vi "Find attached USB cameras.vi"() -> ()   [LabVIEW 2025]
uses:
  <vilib>/userDefined/High Color/IMAQdx.ctl
  <vilib>/nisyscfg/nisyscfg.lvlib
  <resource>/objmgr/nicriosae.rc
  <vilib>/vision/driver/NI_Vision_Acquisition_Software.lvlib
  <resource>/objmgr/imaqdx.rc
panel:
  out "map":map{u32, T1}(c390)
  out "Serial Number":u32[](array[numeric])
  out "Product":string[](array[string])
  out "Camera":string[](array[string])
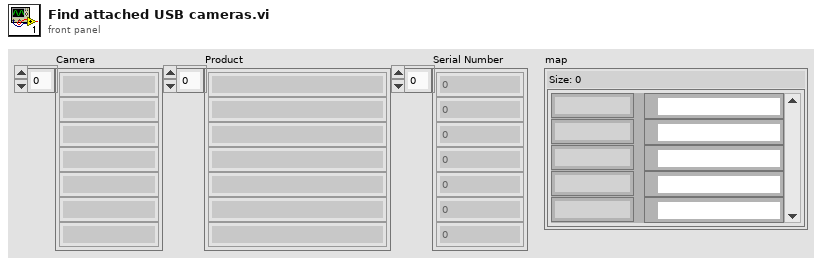
[diagram p1: front panel]
types:
  T1 = typedef "IMAQdx.ctl" = refnum<k21>
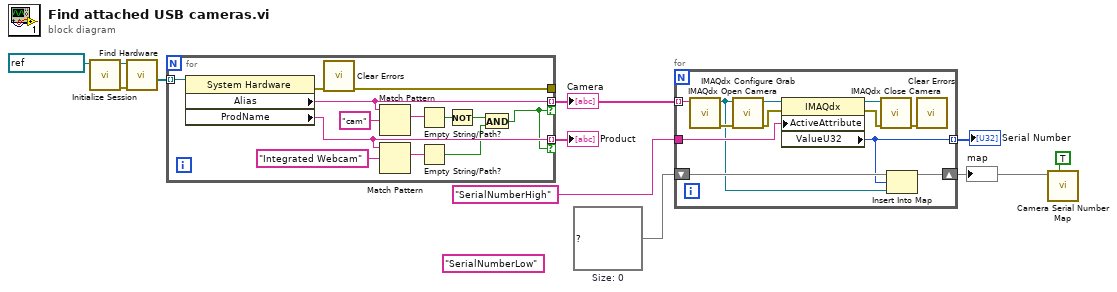
[diagram p0: block diagram]
diagram:
  w4 = map{u32, T1} {}  # Size: 0
  (unwired) "SerialNumberLow"
  n1 = call <vilib>:"Initialize Session.vi"("Target (localhost)"=refnum<k21> "localhost") -> ("error out"=w10:errorcluster, "Session out"=w11:refnum<k21>)  [unwired: 9 in]
  n2 = call <vilib>:"Find Hardware.vi"("error in (no error)"=w10, "Session in"=w11) -> ("Resources out"=w8:refnum<k20>[])  [unwired: 6 in, 3 out]
  n3 = for {
    tunnel: w8 -> [w24] mode=indexing
    tunnel: [w16] -> w7 mode=indexing if=w12
    tunnel: [w22] -> _
    tunnel: [w21] -> w6 mode=indexing if=w12
    n4 = property class="System Hardware"(reference=w24) -> (error out=w23:errorcluster, "Alias"=w21:string, "ProdName"=w16:string)  [unwired: 1 in, 1 out]
    n5 = call <vilib>:"Clear Errors.vi"("error in (no error)"=w23) -> ("error out"=w22:errorcluster)  [unwired: 5 in, 1 out]
    n6 = Match Pattern(string=w21, regular expression="cam") -> (match substring=w19:string)  [unwired: 1 in, 3 out]
    n7 = Match Pattern(string=w16, regular expression="Integrated Webcam") -> (match substring=w15:string)  [unwired: 1 in, 3 out]
    n8 = Empty String/Path?(string/path=w19) -> (empty?=w18:bool)
    n9 = Empty String/Path?(string/path=w15) -> (empty?=w13:bool)
    n10 = Not(x=w18) -> (.not. x?=w14:bool)
    n11 = And(x=w14, y=w13) -> (x .and. y?=w12:bool)
  }
  "Camera" <- w6
  "Product" <- w7
  n12 = for {
    tunnel: w6 -> [w29] mode=indexing
    tunnel: "SerialNumberHigh" -> [w35]
    tunnel: [w27] -> w2 mode=indexing
    shift-right: [w25] -> w3
    shift-left: w4 -> [w28]
    n13 = call <vilib>:"IMAQdx Open Camera.vi"("Session In"=w29) -> ("error out"=w32:errorcluster, "Session Out"=w26:T1)  [unwired: 9 in]
    n14 = call <vilib>:"IMAQdx Configure Grab.vi"("error in"=w32, "Session In"=w26) -> ("error out"=w31:errorcluster, "Session Out"=w36:T1)  [unwired: 8 in]
    n15 = property class="IMAQdx"(reference=w36, error in=w31, "ActiveAttribute"=w35) -> (reference out=w33:T1, error out=w30:errorcluster, "ValueU32"=w27:u32)
    n16 = call <vilib>:"IMAQdx Close Camera.vi"("error in"=w30, "Session In"=w33) -> ("error out"=w34:errorcluster)  [unwired: 9 in]
    n17 = Insert Into Map(map in=w28, key=w27, value=w26) -> (map out=w25:map{u32, T1})  [unwired: 2 out]
    n18 = call <vilib>:"Clear Errors.vi"("error in (no error)"=w34) -> ()  [unwired: 5 in, 2 out]
  }
  "Serial Number" <- w2
  "map" <- w3
  n19 = call "Camera Serial Number Map.vi"("Update"=TRUE, "map"=w3) -> ()  [unwired: 9 in, 1 out]
